vi "SPARK Check Firmware Version.vi"(7 "CAN ID":u8, 8 "error in (no error)":errorcluster, 10 "Firmware Version":T1) -> (0 "error out":errorcluster)   [LabVIEW 2023]
uses:
  Typedef/SPARK Firmware Version.ctl
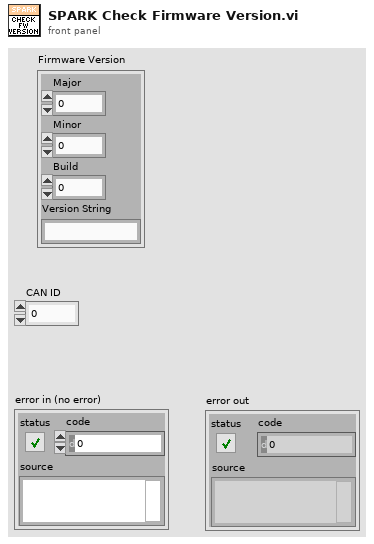
[diagram p1: front panel]
types:
  T1 = typedef "SPARK Firmware Version.ctl" = cluster{"Major":u8, "Minor":u8, "Build":u16, "Version String":string}
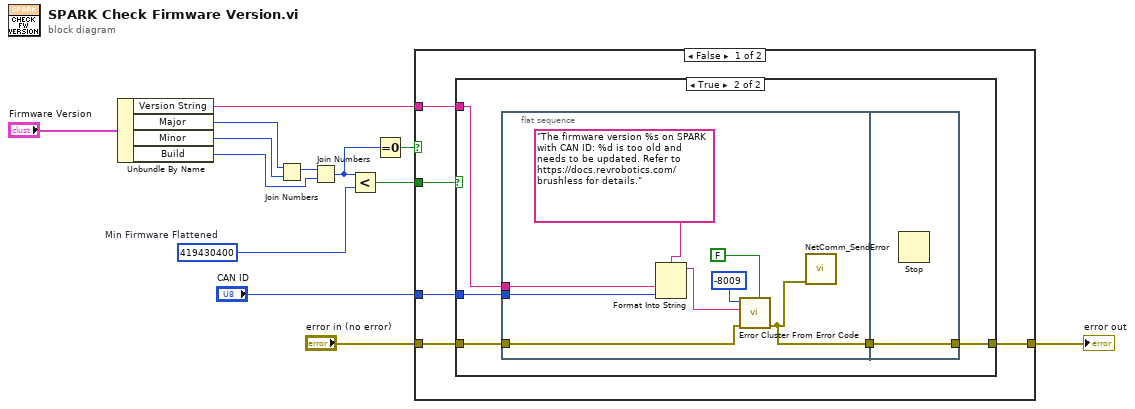
[diagram p0: block diagram]
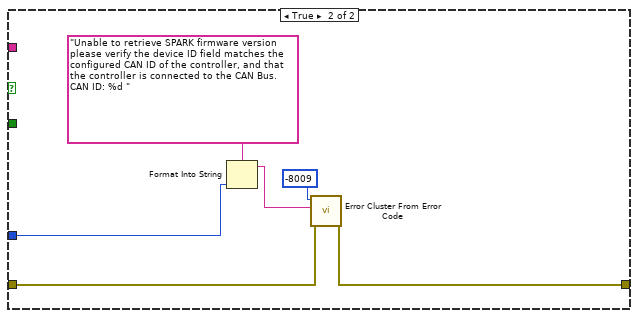
[diagram p3: hidden frame]
diagram:
  w12 = u32 419430400  # Min Firmware Flattened
  n1 = Unbundle By Name("Firmware Version") -> ("Version String"=w1:string, "Major"=w4:u8, "Minor"=w3:u8, "Build"=w2:u16)
  n2 = Join Numbers(hi=w4, lo=w3) -> ((hi.lo)=w13:u16)
  n3 = Join Numbers(hi=w13, lo=w2) -> ((hi.lo)=w11:u32)
  n4 = Less?(x=w11, y=w12) -> (x < y?=w9:bool)
  n5 = Equal To 0?(x=w11) -> (x = 0?=w10:bool)
  n6 = case shown="False" w10 {
    tunnel: w9 -> [w18 _]
    tunnel: "error in (no error)" -> [w17 w39]
    tunnel: [w16 w38] -> w7
    tunnel: w1 -> [w14 _]
    tunnel: "CAN ID" -> [w15 w36]
    frame False {
      n7 = case shown="True" w18 {
        tunnel: w17 -> [w19 w24]
        tunnel: [w19 w21] -> w16
        tunnel: w15 -> [_ w23]
        tunnel: w14 -> [_ w22]
        frame False {
        }
        frame True {
          n8 = flat-sequence {
            tunnel: w24 -> [w29]
            tunnel: w23 -> [w28]
            tunnel: w22 -> [w27]
            tunnel: [w25] -> w20
            tunnel: [w33] -> w21
            tunnel: w20 -> [w33]
            frame #0 {
              n9 = Format Into String(format string="The firmware version %s on SPARK with CAN ID: %d is too old and needs to be updated. Refer to https://docs.revrobotics.com/brushless for details.", w27, w28) -> (resulting string=w32:string)  [unwired: 2 in, 1 out]
              n10 = call <vilib>:"Error Cluster From Error Code.vi"("is warning? (False)"=FALSE, "error in (no error)"=w29, "error message (\"\")"=w32, "error code (0)"=-8009) -> ("error out"=w25:errorcluster)  [unwired: 5 in]
              n11 = call <vilib>:"NetComm_SendError.vi"("error in (no error)"=w25) -> ()  [unwired: 11 in]
            }
            frame #1 {
              n12 = Stop() -> ()  [unwired: 1 in]
            }
          }
        }
      }
    }
    frame True {
      n13 = Format Into String(format string="Unable to retrieve SPARK firmware version please verify the device ID field matches the configured CAN ID of the controller, and that the controller is connected to the CAN Bus. CAN ID: %d ", w36) -> (resulting string=w35:string)  [unwired: 2 in, 1 out]
      n14 = call <vilib>:"Error Cluster From Error Code.vi"("error in (no error)"=w39, "error message (\"\")"=w35, "error code (0)"=-8009) -> ("error out"=w38:errorcluster)  [unwired: 6 in]
    }
  }
  "error out" <- w7
